vi "cXB_trt-1-initni.vi"(8 "err in":errorcluster, 11 "cXB (e)":T1) -> (0 "err out":errorcluster, 3 "cXB (s)":T1)   [LabVIEW 2010]
uses:
  lv_04/commandes/cX.ctl
  lv_04/commandes/cSTA_varid.ctl
  lv_04/commandes/c_TDMS_ch_variable.ctl
  lv_04/commandes/c_TDMS_ch_donnees.ctl
  lv_04/commandes/c0-var-n.ctl
  lv_04/commandes/cSTA_num_do_cr.ctl
  lv_04/commandes/c02-do-num.ctl
  lv_04/commandes/c04-stat-num.ctl
  lv_04/commandes/cSTA_txt_do_cr.ctl
  lv_04/commandes/c02-do-txt.ctl
  lv_04/commandes/c04-stat-txt.ctl
  lv_04/commandes/cSTA_dist.ctl
  lv_04/commandes/c03-dist-S.ctl
  lv_04/commandes/c0-dist-xy.ctl
  lv_04/commandes/c03-dist-T.ctl
  lv_04/commandes/c03-dist-SPC.ctl
  lv_02/MIF_N_txt-de-obs.vi
  lv_02/MIF_N_num_cont-de-obs.vi
  lv_02/lv_02.lvlib
  lv_04/lv_04.lvlib
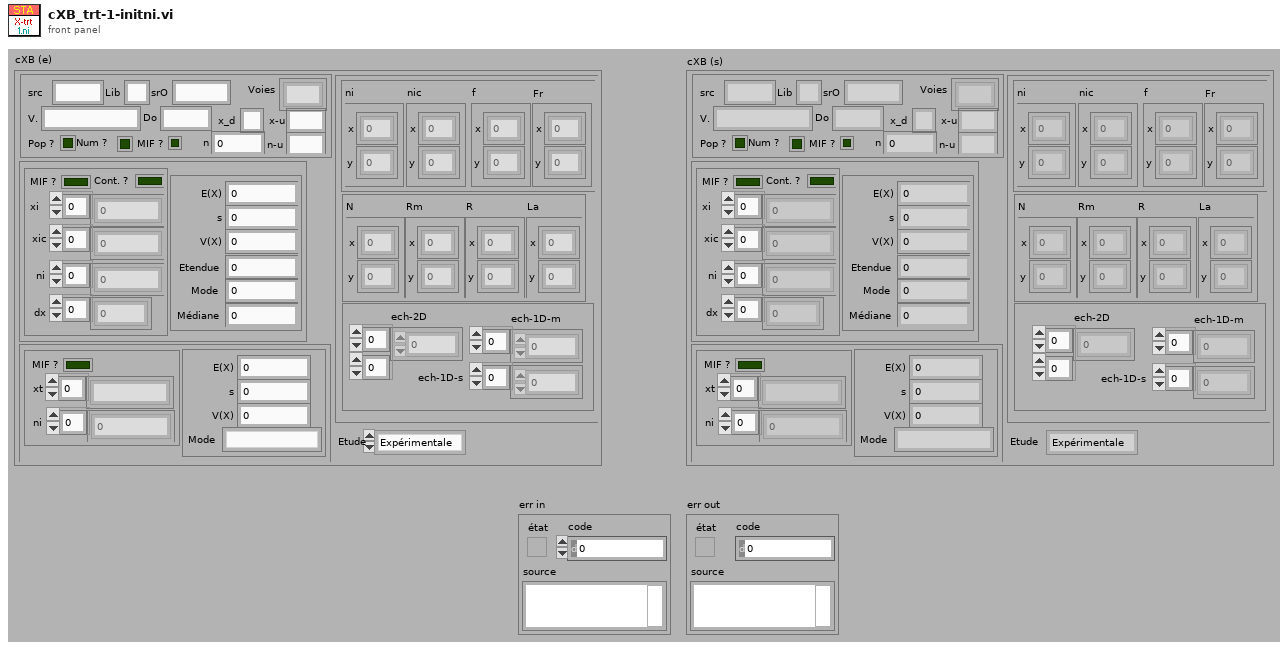
[diagram p1: front panel]
types:
  T1 = typedef "lv_04.lvlib/cX.ctl" = cluster{"src":T2, "num":T6, "txt":T9, "dist":T12, "Etude":enum16{"Expérimentale", "Modèle"}}
  T2 = typedef "lv_04.lvlib/cSTA_varid.ctl" = cluster{"src":string, "Lib":string, "srO":string, "V.":T3, "Voies":string[], "Do":T4, "n":T5, "Num ?":bool, "Pop ?":bool, "x_d":string, "x-u":string, "n-u":string, "MIF ?":bool}
  T3 = typedef "lv_04.lvlib/c_TDMS_ch_variable.ctl" = string
  T4 = typedef "lv_04.lvlib/c_TDMS_ch_donnees.ctl" = string
  T5 = typedef "lv_04.lvlib/c0-var-n.ctl" = i32
  T6 = typedef "lv_04.lvlib/cSTA_num_do_cr.ctl" = cluster{"do":T7, "sta":T8}
  T7 = typedef "lv_04.lvlib/c02-do-num.ctl" = cluster{"MIF ?":bool, "Cont. ?":bool, "xi":dbl[], "xic":dbl[], "ni":u32[], "dx":dbl[]}
  T8 = typedef "lv_04.lvlib/c04-stat-num.ctl" = cluster{"E(X)":dbl, "s":dbl, "V(X) ":dbl, "Etendue":dbl, "Mode":dbl, "Médiane":dbl}
  T9 = typedef "lv_04.lvlib/cSTA_txt_do_cr.ctl" = cluster{"do":T10, "sta":T11}
  T10 = typedef "lv_04.lvlib/c02-do-txt.ctl" = cluster{"xt":string[], "ni":dbl[], "MIF ?":bool}
  T11 = typedef "lv_04.lvlib/c04-stat-txt.ctl" = cluster{"E(X)":dbl, "s":dbl, "V(X) ":dbl, "Mode":string}
  T12 = typedef "lv_04.lvlib/cSTA_dist.ctl" = cluster{"S":T13, "T":T15, "spc":T16}
  T13 = typedef "lv_04.lvlib/c03-dist-S.ctl" = cluster{"nic":T14, "f":T14, "Fr":T14, "ni":T14}
  T14 = typedef "lv_04.lvlib/c0-dist-xy.ctl" = cluster{"x":dbl[], "y":dbl[]}
  T15 = typedef "lv_04.lvlib/c03-dist-T.ctl" = cluster{"N":T14, "Rm":T14, "R":T14, "La":T14}
  T16 = typedef "lv_04.lvlib/c03-dist-SPC.ctl" = cluster{"ech-2D":dbl[][], "ech-1D-m":dbl[], "ech-1D-s":dbl[]}
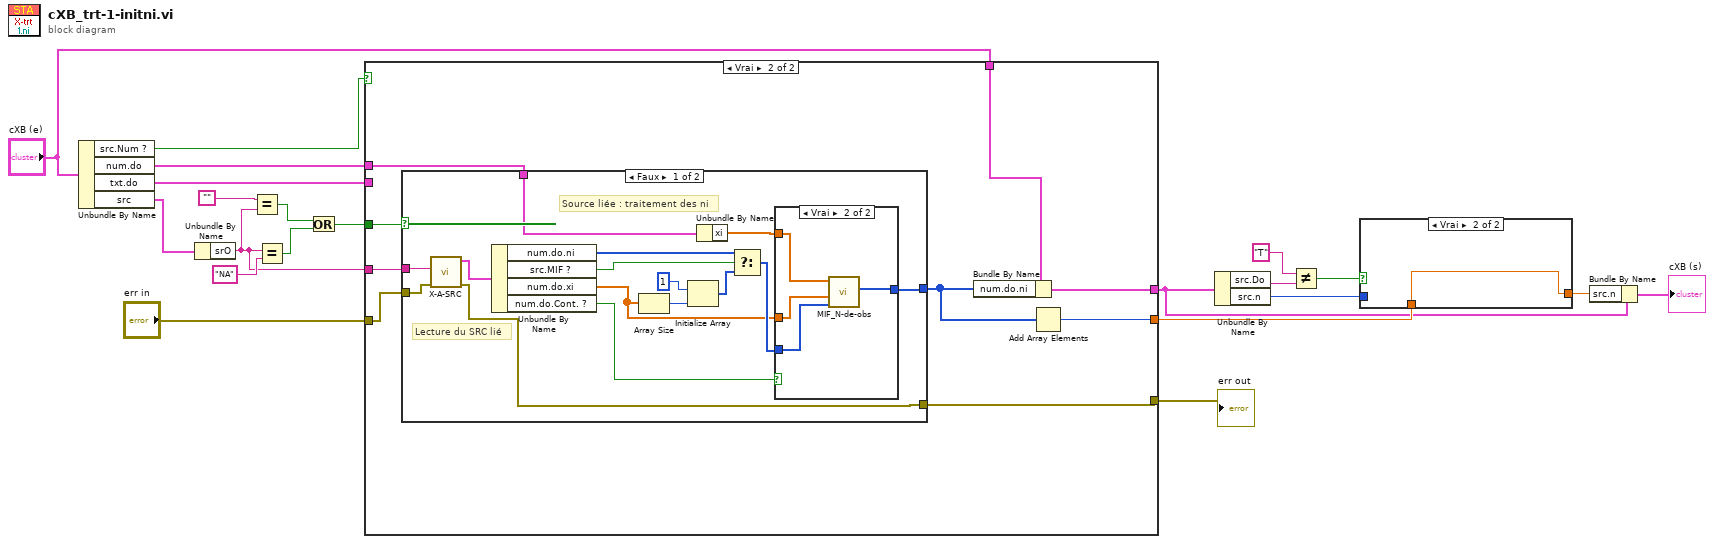
[diagram p0: block diagram]
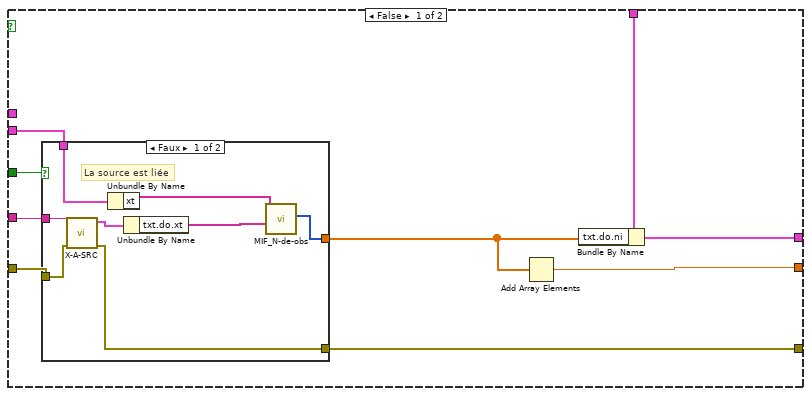
[diagram p3: hidden frame]
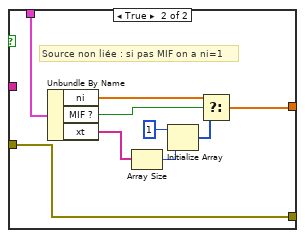
[diagram p4: hidden frame]
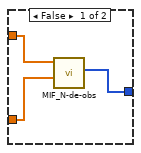
[diagram p5: hidden frame]
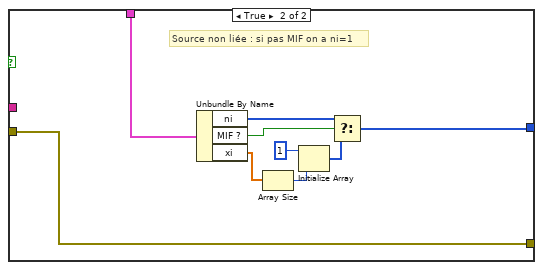
[diagram p6: hidden frame]
diagram:
  n1 = Unbundle By Name("cXB (e)") -> ("src.Num ?"=w14:bool, "num.do"=w12:T7, "txt.do"=w11:T10, "src"=w13:T2)
  n2 = Unbundle By Name(w13) -> ("srO"=w19:string)
  n3 = Equal?(x="", y=w19) -> (x = y?=w17:bool)
  n4 = Equal?(x=w19, y="NA") -> (x = y?=w16:bool)
  n5 = Or(x=w17, y=w16) -> (x .or. y?=w15:bool)
  n6 = case shown="Vrai" w14 {
    tunnel: [w26 w51] -> w1
    tunnel: "err in" -> [w28 w56]
    tunnel: w19 -> [w30 w55]
    tunnel: w15 -> [w29 w54]
    tunnel: w12 -> [_ w52]
    tunnel: w11 -> [w27 _]
    tunnel: "cXB (e)" -> [w25 w50]
    tunnel: [w24 w53] -> w9
    tunnel: [w22 w48] -> w3
    frame False {
      n7 = case shown="Faux" w29 {
        tunnel: w27 -> [w38 w41]
        tunnel: [w35 w40] -> w23
        tunnel: w30 -> [w34 _]
        tunnel: w28 -> [w33 w39]
        tunnel: [w32 w39] -> w24
        frame False {
          # "La source est liée"
          n8 = call "X-A-SRC.vi"("err in"=w33, "src-nom"=w34) -> ("err out"=w32:errorcluster, "SRC-X (s)"=w31:T1)  [unwired: 8 in]
          n9 = Unbundle By Name(w38) -> ("xt"=w37:string[])
          n10 = Unbundle By Name(w31) -> ("txt.do.xt"=w36:string[])
          n11 = call-poly "MIF_N-de-obs.vi"("xt obs"=w36, "xt mif"=w37) -> ("ni-mif"=w35:i32[])  [unwired: 9 in]
        }
        frame True {
          # "Source non liée : si pas MIF on a ni=1"
          n12 = Unbundle By Name(w41) -> ("ni"=w46:dbl[], "MIF ?"=w45:bool, "xt"=w42:string[])
          n13 = Array Size(array=w42) -> (size(s)=w44:i32)
          n14 = Initialize Array(1 ("x_deb"), w44) -> (w47:i32[])
          n15 = Select(t=w46, s=w45, f=w47) -> (s? t:f=w40:dbl[])
        }
      }
      n16 = Add Array Elements(numeric array=w23) -> (sum=w22:dbl)
      n17 = Bundle By Name(cluster=w25, "txt.do.ni"=w23) -> (w26:T1)
    }
    frame True {
      n18 = case shown="Faux" w54 {
        tunnel: w52 -> [w63 w81]
        tunnel: [w64 w80] -> w49
        tunnel: w55 -> [w60 _]
        tunnel: w56 -> [w59 w79]
        tunnel: [w58 w79] -> w53
        frame False {
          # "Lecture du SRC lié"
          # "Source liée : traitement des ni"
          n19 = call "X-A-SRC.vi"("err in"=w59, "src-nom"=w60) -> ("err out"=w58:errorcluster, "SRC-X (s)"=w57:T1)  [unwired: 8 in]
          n20 = Unbundle By Name(w57) -> ("num.do.ni"=w70:u32[], "src.MIF ?"=w69:bool, "num.do.xi"=w66:dbl[], "num.do.Cont. ?"=w62:bool)
          n21 = Array Size(array=w66) -> (size(s)=w65:i32)
          n22 = Initialize Array(1 ("x_deb"), w65) -> (w71:i32[])
          n23 = Unbundle By Name(w63) -> ("xi"=w61:dbl[])
          n24 = Select(t=w70, s=w69, f=w71) -> (s? t:f=w67:u32[])
          n25 = case shown="Vrai" w62 {
            tunnel: [w72 w75] -> w64
            tunnel: w66 -> [w73 w77]
            tunnel: w67 -> [_ w76]
            tunnel: w61 -> [w74 w78]
            frame False {
              n26 = call-poly "MIF_N-de-obs.vi"("X-OBS"=w73, "Xi-classes"=w74) -> ("N-MIF"=w72:u32[])  [unwired: 9 in]
            }
            frame True {
              n27 = call-poly "MIF_N-de-obs.vi"("ni-OBS"=w76, "X-OBS"=w77, "Xi-classes"=w78) -> ("N-MIF"=w75:u32[])  [unwired: 8 in]
            }
          }
        }
        frame True {
          # "Source non liée : si pas MIF on a ni=1"
          n28 = Unbundle By Name(w81) -> ("ni"=w86:u32[], "MIF ?"=w85:bool, "xi"=w82:dbl[])
          n29 = Array Size(array=w82) -> (size(s)=w84:i32)
          n30 = Initialize Array(1 ("x_deb"), w84) -> (w87:i32[])
          n31 = Select(t=w86, s=w85, f=w87) -> (s? t:f=w80:u32[])
        }
      }
      n32 = Bundle By Name(cluster=w50, "num.do.ni"=w49) -> (w51:T1)
      n33 = Add Array Elements(numeric array=w49) -> (sum=w48:u32)
    }
  }
  "err out" <- w9
  n34 = Unbundle By Name(w1) -> ("src.Do"=w8:T4, "src.n"=w5:T5)
  n35 = Not Equal?(x=T4 "T", y=w8) -> (x != y?=w6:bool)
  n36 = case shown="Vrai" w6 {
    tunnel: w5 -> [w88 _]
    tunnel: [w88 w89] -> w4
    tunnel: w3 -> [_ w89]
    frame False {
    }
    frame True {
    }
  }
  n37 = Bundle By Name(cluster=w1, "src.n"=w4) -> (→"cXB (s)":T1)
